vi "Create_DVR.vi"(8 "error in (no error)":errorcluster, 11 "EVE in":refnum<class "EVE.lvclass">) -> (0 "error out":errorcluster, 3 "EVE reference":refnum<data-value>)   [LabVIEW 2013, in "EVE.lvclass"]
uses:
  EVE.lvclass
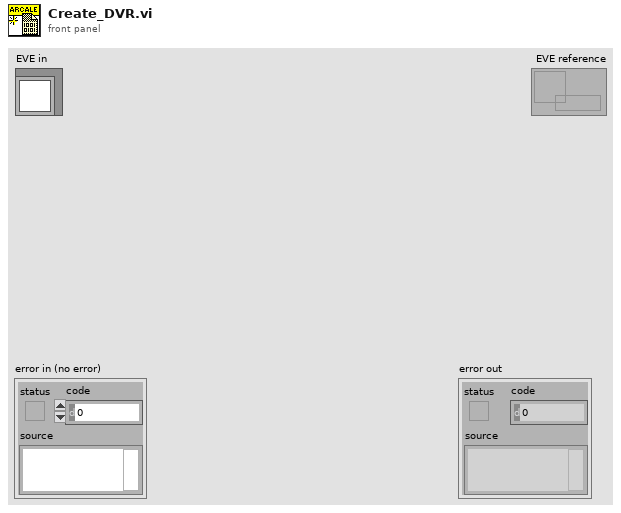
[diagram p1: front panel]
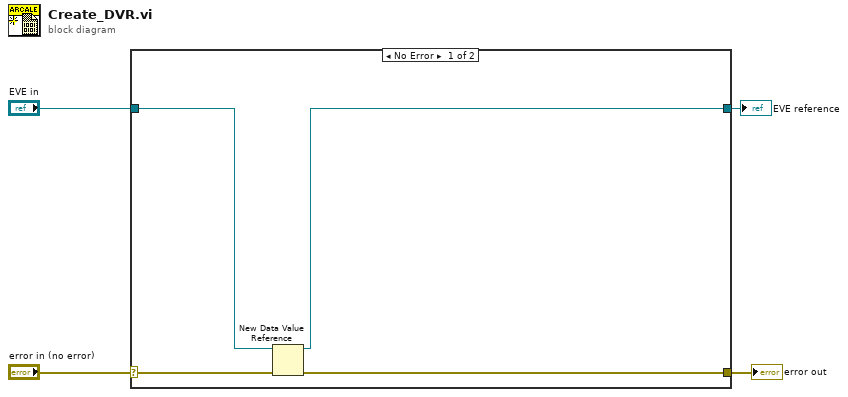
[diagram p0: block diagram]
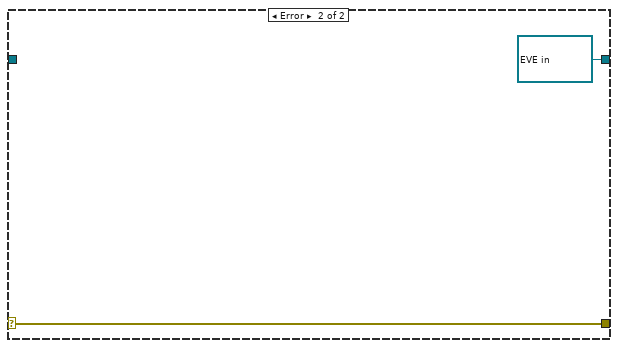
[diagram p2: hidden frame]
diagram:
  n1 = case shown="No Error" "error in (no error)" {
    selector: "error in (no error)" -> [w8 w10]
    tunnel: [w7 w10] -> w3
    tunnel: [w6 refnum<data-value> refnum ("data value reference")] -> w1
    tunnel: "EVE in" -> [w5 _]
    frame No Error {
      n2 = New Data Value Reference(data value=w5, error in=w8) -> (data value reference=w6:refnum<data-value>, error out=w7:errorcluster)
    }
    frame Error {
    }
  }
  "error out" <- w3
  "EVE reference" <- w1
